vi "tm3samp_09_wview_wVision.vi"() -> ()   [LabVIEW 2023]
panel:
  out "Display":T1(plugin-control)
  in  "Vertical Width":i32=512
  in  "Horizontal Width":i32=512
  in  "Vertical Offset B":i32=64
  in  "Horizontal Offset B":i32=256
  in  "Vertical Offset A":i32=128
  in  "Horizontal Offset A":i32=512
  out "Frames Per Second":dbl
  in  "Quit":bool
  out "Error Out":errorcluster {"code" format="%.0x"}
  # "This is just a simple example\nof how to setup a camera for\na W-View application with\na Flash4.0 LT"
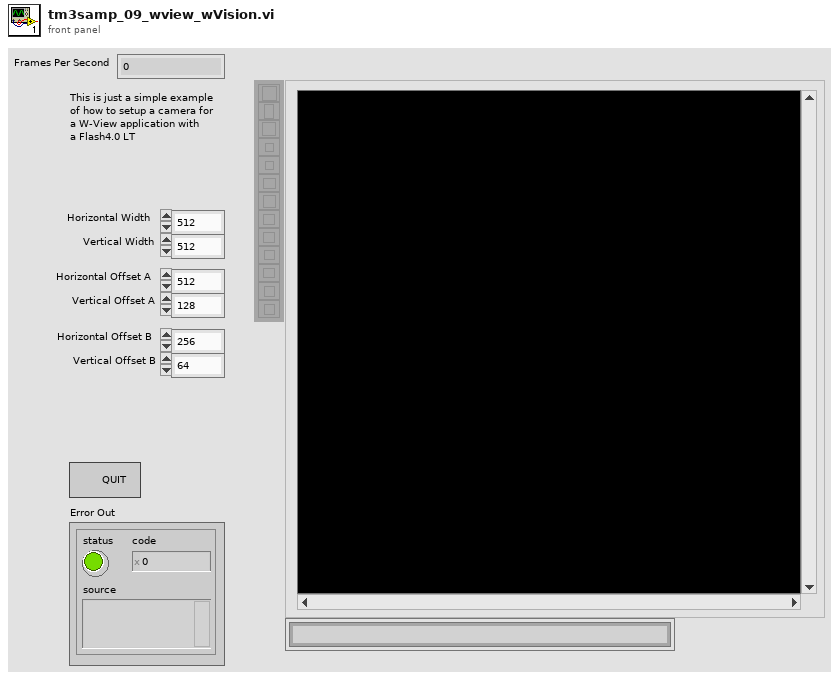
[diagram p1: front panel]
types:
  T1 = typedef "IMAQ Image.ctl" = refnum<image>
  T2 = typedef "Image Type" = u32
  T3 = cluster{"Horizontal Offset A":i32, "Vertical Offset A":i32, "Horizontal Offset B":i32, "Vertical Offset B":i32, "Horizontal Width":i32, "Vertical Width":i32}
  T4 = cluster{"height":u32, "width":u32, "datatype":u32}
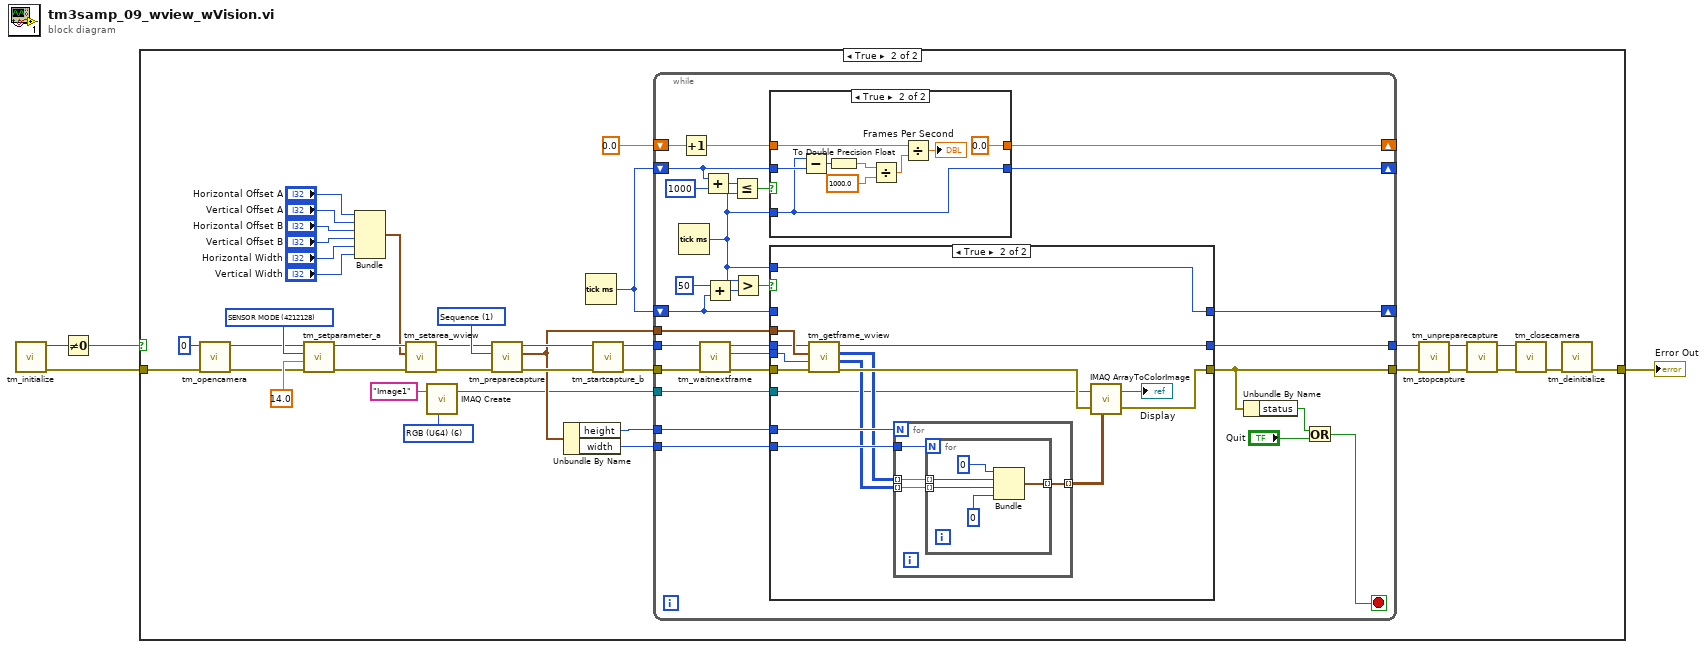
[diagram p0: block diagram]
diagram:
  n1 = call "tm_initialize.vi"() -> ("error out"=w1:errorcluster, "Number Of Cameras"=w2:u32)  [unwired: 8 in, 2 out]
  n2 = Not Equal To 0?(x=w2) -> (x != 0?=w4:bool)
  n3 = case shown="True" w4 {
    tunnel: w1 -> [w5 w43]
    tunnel: [w5 w40] -> w3
    frame False {
    }
    frame True {
      w9 = T2 6 items=["Grayscale (U8)", "Grayscale (I16)", "Grayscale (SGL)", "Complex (CSG)", "RGB (U32)", "HSL (U32)", "RGB (U64)", "Grayscale (U16)"] ("Image Type")
      w25 = u32 4212128 items=["SENSOR MODE"=4212128, "CCD MODE"=4212384, "READOUT MODE"=4211872, "ACTIVE VIEW INDEX"=4343136, "BITS PER CHANNEL"=4342976, "IMAGE PIXEL TYPE"=4343296, "BINNING"=4215968, "EXPOSURE TIME"=2049184, "CONTRAST GAIN"=3163312, "CONTRAST OFFSET"=3163328, "LIGHT MODE"=2114720, "SENSITIVITY"=2114992, "PHOTON IMAGING MODE"=2115200, "HIGH DYNAMIC RANGE MODE"=3163360, "WHITE BALANCE"=3163568, "TEMPERATURE"=2115232, "TEMPERATURE TARGET"=2115264, "SENSOR COOLER FAN"=2115296, "LINEBUNDLE HEIGHT"=4212192, "MECHANICAL SHUTTER"=2115488, "BACK FOCUS POSITION"=8422304, "TRIGGER CONNECTOR"=1066432, "TRIGGER SOURCE"=1066144, "OUTPUT TRIGGER SOURCE"=1852576, "TRIGGER GLOBAL EXPOSURE"=2049680, "FIRST TRIGGER BEHAVIOR"=2049696, "CHANNEL SYNC"=1852352, "READOUT DIRECTION"=4211904, "PRE HSYNC COUNT"=1852704, "INTERNAL LINE SPEED"=4191408, "INTERNAL LINE INTERVAL"=4191424] ("Parameter")
      w31 = 1 items=["Snap", "Sequence"] ("Capture mode")
      n4 = call "tm_opencamera.vi"("error in (no error)"=w43, "Camera Index"=u32 0) -> ("error out"=w23:errorcluster, "Handle out"=w24:u32)  [unwired: 7 in, 1 out]
      n5 = call "tm_setparameter_a.vi"("error in (no error)"=w23, "Value in"=14.0, "Parameter"=w25, "Handle in"=w24) -> ("error out"=w21:errorcluster, "Handle out"=w22:u32)  [unwired: 6 in]
      n6 = Bundle("Horizontal Offset A"="Horizontal Offset A", "Vertical Offset A"="Vertical Offset A", "Horizontal Offset B"="Horizontal Offset B", "Vertical Offset B"="Vertical Offset B", "Horizontal Width"="Horizontal Width", "Vertical Width"="Vertical Width") -> (w18:T3)  [unwired: 1 in]
      n7 = call "tm_setarea_wview.vi"("error in (no error)"=w21, "Sub Region"=w18, "Handle in"=w22) -> ("error out"=w20:errorcluster, "Handle out"=w19:u32)  [unwired: 7 in]
      n8 = call "IMAQ Create"("Image Name"="Image1", "Image Type"=w9) -> ("New Image"=w8:T1)  [unwired: 3 in, 1 out]
      n9 = call "tm_preparecapture.vi"("error in (no error)"=w20, "Capture mode"=w31, "Handle in"=w19) -> ("error out"=w29:errorcluster, "Buffer Info"=w11:T4, "Handle out"=w30:u32)  [unwired: 5 in, 1 out]
      n10 = Unbundle By Name(w11) -> ("height"=w7:u32, "width"=w6:u32)
      n11 = Tick Count (ms)() -> (millisecond timer value=w27:u32)
      n12 = call "tm_startcapture_b.vi"("error in (no error)"=w29, "Handle in"=w30) -> ("error out"=w32:errorcluster, "Handle out"=w33:u32)  [unwired: 8 in]
      n13 = while {
        tunnel: [w50] -> w36
        tunnel: [w51] -> w37
        tunnel: w11 -> [w48]
        tunnel: w33 -> [w68]
        tunnel: w32 -> [w69]
        shift-right: [w66] -> _
        shift-left: w27 -> [w63]
        shift-right: [w67] -> _
        shift-left: 0.0 -> [w60]
        shift-right: [w49] -> _
        shift-left: w27 -> [w52]
        tunnel: w7 -> [w47]
        tunnel: w6 -> [w46]
        tunnel: w8 -> [w45]
        stop <- w44 stop-if-true
        n14 = Tick Count (ms)() -> (millisecond timer value=w53:u32)
        n15 = Increment(x=w60) -> (x+1=w61:dbl)
        n16 = call "tm_waitnextframe.vi"("error in (no error)"=w69, "Handle in"=w68) -> ("error out"=w58:errorcluster, "Frame Index"=w57:i32, "Handle out"=w59:u32)  [unwired: 6 in, 1 out]
        n17 = Add(x=w63, y=u32 1000) -> (x+y=w65:u32)
        n18 = Add(x=u32 50, y=w52) -> (x+y=w55:u32)
        n19 = Less Or Equal?(x=w65, y=w53) -> (x <= y?=w62:bool)
        n20 = Greater?(x=w53, y=w55) -> (0:w54:bool)
        n21 = case shown="True" w62 {
          tunnel: w63 -> [w100 w103]
          tunnel: [w100 w101] -> w66
          tunnel: w61 -> [w99 w107]
          tunnel: w53 -> [_ w101]
          tunnel: [w99 0.0] -> w67
          frame False {
          }
          frame True {
            n22 = Subtract(x=w101, y=w103) -> (x-y=w102:u32)
            n23 = To Double Precision Float(number=w102) -> (double precision float=w109:dbl)
            n24 = Divide(x=w109, y=1000.0) -> (x/y=w106:dbl)
            n25 = Divide(x=w107, y=w106) -> (x/y=→"Frames Per Second":dbl)
          }
        }
        n26 = case shown="True" w54 {
          tunnel: w59 -> [w74 w85]
          tunnel: w58 -> [w73 w88]
          tunnel: w57 -> [_ w87]
          tunnel: w52 -> [w72 _]
          tunnel: w53 -> [_ w89]
          tunnel: [w74 w84] -> w50
          tunnel: [w73 w76] -> w51
          tunnel: [w72 w89] -> w49
          tunnel: w48 -> [_ w86]
          tunnel: w47 -> [_ w82]
          tunnel: w46 -> [_ w81]
          tunnel: w45 -> [_ w75]
          frame False {
          }
          frame True {
            n27 = call "tm_getframe_wview.vi"("error in (no error)"=w88, "Frame Index"=w87, "Buffer Info"=w86, "Handle in"=w85) -> ("error out"=w83:errorcluster, "Data B"=w79:u16[][], "Data A"=w80:u16[][], "Handle out"=w84:u32)  [unwired: 3 in, 1 out]
            n28 = for {
              N: w82 -> [_]
              tunnel: w81 -> [w93]
              tunnel: w80 -> [w92] mode=indexing
              tunnel: w79 -> [w91] mode=indexing
              tunnel: [w90] -> w78 mode=indexing
              n29 = for {
                N: w93 -> [_]
                tunnel: w92 -> [w96] mode=indexing
                tunnel: w91 -> [w95] mode=indexing
                tunnel: [w97] -> w90 mode=indexing
                n30 = Bundle(u16 0, "Numeric"=w96, "Numeric"=w95, u16 0) -> (w97:cluster{u16, "Numeric":u16, "Numeric":u16, u16})  [unwired: 1 in]
              }
            }
            n31 = call "IMAQ ArrayToColorImage"("Image"=w75, "Image Pixels (U64)"=w78, "error in (no error)"=w83) -> ("Image Out"=→"Display":T1, "error out"=w76:errorcluster)  [unwired: 2 in]
          }
        }
        n32 = Unbundle By Name(w51) -> ("status"=w71:bool)
        n33 = Or(x=w71, y="Quit") -> (x .or. y?=w44:bool)
      }
      n34 = call "tm_stopcapture.vi"("error in (no error)"=w37, "Handle in"=w36) -> ("error out"=w34:errorcluster, "Handle out"=w35:u32)  [unwired: 8 in]
      n35 = call "tm_unpreparecapture.vi"("error in (no error)"=w34, "Handle in"=w35) -> ("error out"=w39:errorcluster, "Handle out"=w38:u32)  [unwired: 8 in]
      n36 = call "tm_closecamera.vi"("error in (no error)"=w39, "Handle in"=w38) -> ("error out"=w41:errorcluster)  [unwired: 9 in]
      n37 = call "tm_deinitialize.vi"("error in (no error)"=w41) -> ("error out"=w40:errorcluster)  [unwired: 10 in]
    }
  }
  "Error Out" <- w3
